vi "打开子VI.vi"(9 "窗口大小":cluster{"wide":i32, "Top":i32} caption="VI大小", 10 "窗口位置":T1 caption="VI位置", 11 "引用":refnum<vi>) -> (0 "错误输出":errorcluster, 3 "引用输出":refnum<vi>)   [LabVIEW 2018]
uses:
  <vilib>/Utility/miscctls.llb/LVPositionTypeDef.ctl
  <vilib>/Utility/miscctls.llb/LVRectTypeDef.ctl
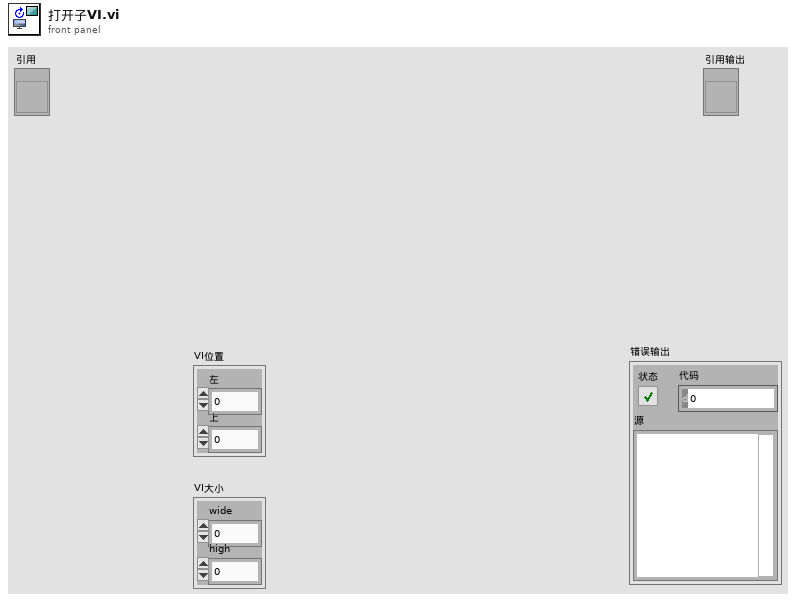
[diagram p1: front panel]
types:
  T1 = typedef "LVPositionTypeDef.ctl" = cluster{"Left":i32, "Top":i32}
  T2 = typedef "LVRectTypeDef.ctl" = cluster{"Left":i16, "Top":i16, "Right":i16, "Bottom":i16}
  T3 = enum32{"Bad", "Idle", "Run top level", "Running"}
  T4 = enum32{"Invalid", "Standard", "Closed", "Hidden", "Minimized", "Maximized"}
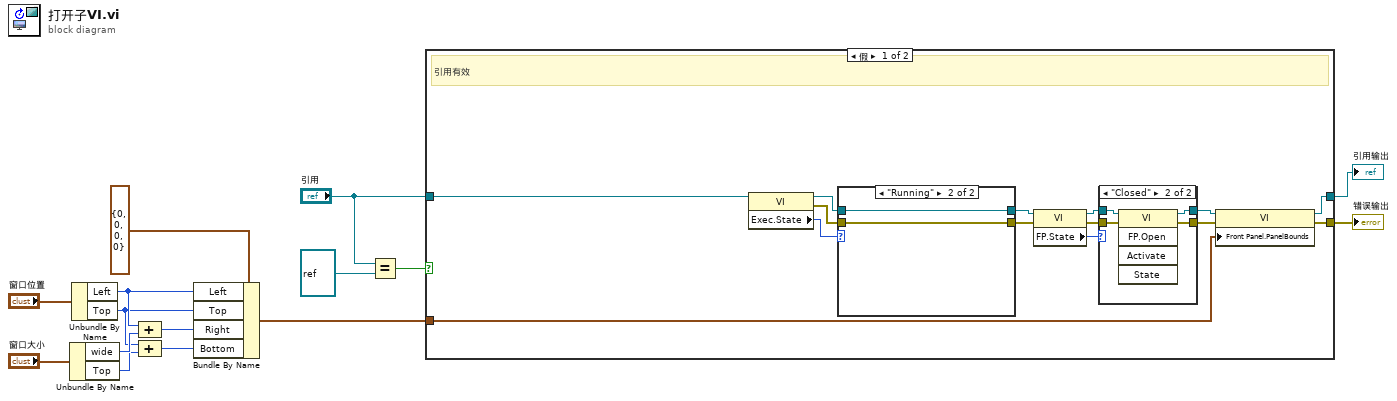
[diagram p0: block diagram]
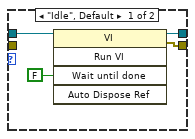
[diagram p3: hidden frame]
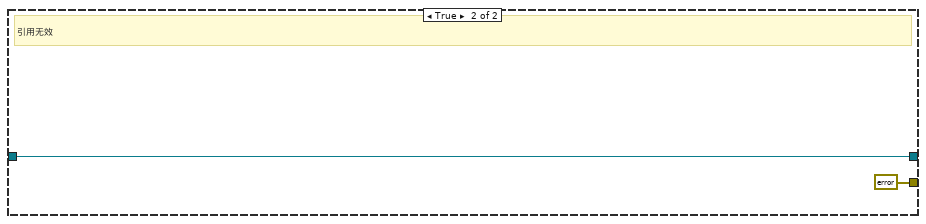
[diagram p4: hidden frame]
diagram:
  n1 = Unbundle By Name("窗口大小") -> ("wide"=w10:i32, "Top"=w9:i32)
  n2 = Unbundle By Name("窗口位置") -> ("Left"=w8:i32, "Top"=w7:i32)
  n3 = Compound Arithmetic op=ADD(w8, w10) -> (w13:i32)
  n4 = Compound Arithmetic op=ADD(w7, w9) -> (w12:i32)
  n5 = Bundle By Name(cluster=T2 {"Left"=0, "Top"=0, "Right"=0, "Bottom"=0} ("前面板窗口:前面板边界"), "Left"=w8, "Top"=w7, "Right"=w13, "Bottom"=w12) -> (w5:T2)
  n6 = Equal?(x="引用", y=refnum<vi> refnum ("引用")) -> (x = y?=w2:bool)
  n7 = case shown="假" w2 {
    tunnel: [w27 errorcluster {"status"=FALSE, "code"=0, "source"=""} ("error out")] -> w15
    tunnel: w5 -> [w26 _]
    tunnel: [w25 w43] -> w4
    tunnel: "引用" -> [w16 w43]
    frame False {
      # "引用有效"
      n8 = property class="VI"(reference=w16) -> (reference out=w24:refnum<vi>, error out=w22:errorcluster, "Exec.State"=w23:T3)  [unwired: 1 in]
      n9 = case shown="\"Running\"" w23 {
        tunnel: [w39 w41] -> w21
        tunnel: [w38 w40] -> w20
        tunnel: w24 -> [w36 w41]
        tunnel: w22 -> [_ w40]
        frame "Idle", Default {
          n10 = invoke class="VI" method="Run VI"(reference=w36, "Wait until done"=FALSE ("结束前等待")) -> (reference out=w39:refnum<vi>, error out=w38:errorcluster)  [unwired: 3 in, 3 out]
        }
        frame "Running" {
        }
      }
      n11 = property class="VI"(reference=w21, error in=w20) -> (reference out=w19:refnum<vi>, error out=w17:errorcluster, "FP.State"=w18:T4)
      n12 = case shown="\"Closed\"" w18 {
        tunnel: [w31 w35] -> w29
        tunnel: [w30 w34] -> w28
        tunnel: w19 -> [w31 w33]
        tunnel: w17 -> [w30 w32]
        frame "Standard", Default {
        }
        frame "Closed" {
          n13 = invoke class="VI" method="FP.Open"(reference=w33, error in=w32) -> (reference out=w35:refnum<vi>, error out=w34:errorcluster)  [unwired: 3 in, 3 out]
        }
      }
      n14 = property class="VI"(reference=w29, error in=w28, "Front Panel.PanelBounds"=w26) -> (reference out=w25:refnum<vi>, error out=w27:errorcluster)
    }
    frame True {
      # "引用无效"
    }
  }
  "错误输出" <- w15
  "引用输出" <- w4
